vi "sv_Uniquify Existing Group Name.vi"(0 "tdms file ref":refnum<k34>, 5 "group name":string, 11 "error in":errorcluster) -> (4 "tdms file out":refnum<k34>, 6 "unique group":string, 15 "error out":errorcluster)   [LabVIEW 2017]
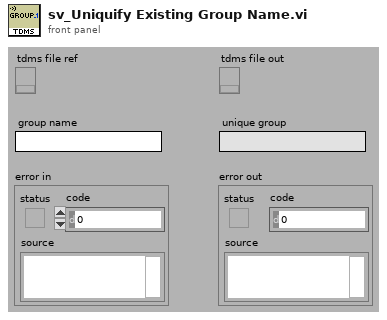
[diagram p1: front panel]
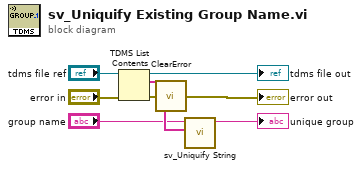
[diagram p0: block diagram]
diagram:
  n1 = TDMS List Contents(4:"error in", 7:"tdms file ref") -> (0:w1:errorcluster, 2:w8:string[], 3:→"tdms file out":refnum<k34>)  [unwired: 1 in, 1 out]
  n2 = call <vilib>:"ClearError.vi"("error in (no error)"=w1) -> ("error out"=→"error out":errorcluster)
  n3 = call <vilib>:"sv_Uniquify String.vi"("reserved strings"=w8, "string"="group name") -> ("unique string"=→"unique group":string)  [unwired: 7 in, 2 out]
